vi "Savecalil_data.vi"(8 "错误输入（无错误）":errorcluster, 11 "PDLSTS":refnum<k24>) -> (0 "错误输出":errorcluster)   [LabVIEW 2017]
doc: "// Save Calculated IL (Cancel for SOP wavelength dependence)\n // This method must be run after the PDL Calculation"
uses:
  D:/test/PDLSTS/LV_PDL_Sample/DLL/STSProcess.dll
  DLL/STSProcess.dll
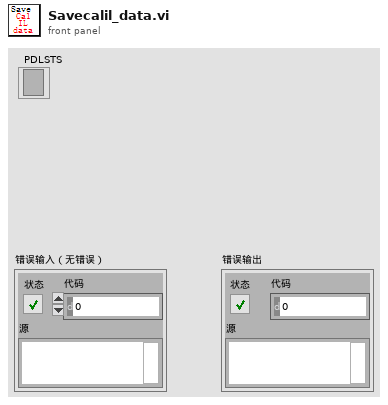
[diagram p1: front panel]
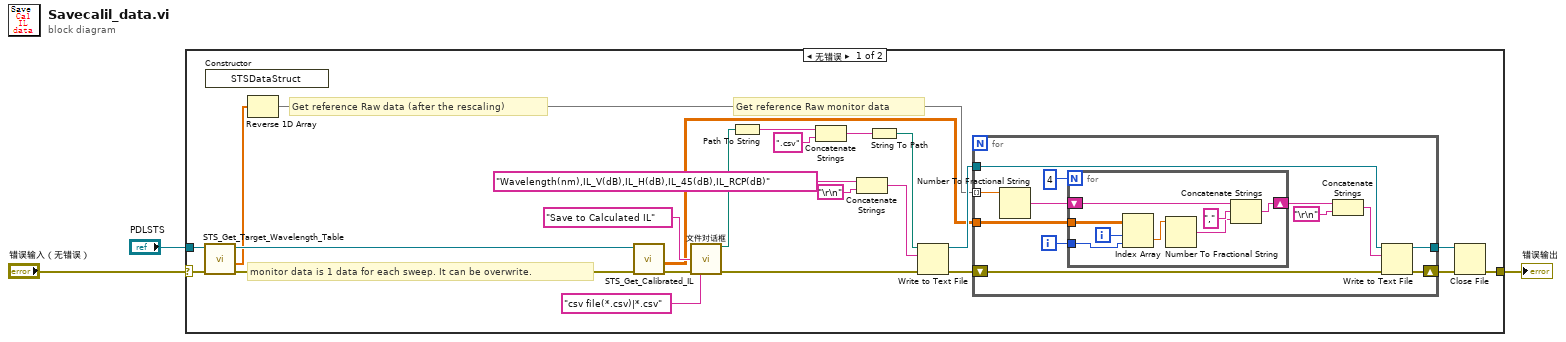
[diagram p0: block diagram]
diagram:
  n1 = case shown="无错误" "错误输入（无错误）" {
    selector: "错误输入（无错误）" -> [w26 w48]
    tunnel: [w27 w48] -> w3
    tunnel: "PDLSTS" -> [w25 _]
    frame No Error {
      # "Get reference Raw monitor data"
      # "monitor data is 1 data for each sweep. It can be overwrite."
      # "Get reference Raw data (after the rescaling)"
      n2 = call "STS_Get_Target_Wavelength_Table.vi"("错误输入（无错误）"=w26, ".NET引用句柄输入"=w25) -> ("error out"=w10:errorcluster, "wavelengths"=w5:dbl[], "引用输出"=w11:refnum<k24>)  [unwired: 7 in]
      n3 = constructor class="STSDataStruct"() -> ()  [unwired: 3 in, 3 out]
      n4 = Reverse 1D Array(array=w5) -> (reversed array=w4:dbl[])
      n5 = call "STS_Get_Calibrated_IL.vi"("错误输入（无错误）"=w10, ".NET引用句柄输入"=w11) -> ("error out"=w8:errorcluster, "calibratedIL"=w6:sgl[][])  [unwired: 7 in, 1 out]
      n6 = call "文件对话框"("default name"="Save to Calculated IL" ("字符串"), "error in"=w8, "pattern (all files)"="csv file(*.csv)|*.csv") -> ("selected path"=w13:path, "error out"=w21:errorcluster)  [unwired: 9 in, 2 out]
      n7 = Path To String(path=w13) -> (string=w12:string)
      n8 = Concatenate Strings(w12, ".csv" ("名称或相对路径")) -> (w19:string)
      n9 = Concatenate Strings("Wavelength(nm),IL_V(dB),IL_H(dB),IL_45(dB),IL_RCP(dB)", "\r\n") -> (w23:string)
      n10 = String To Path(string=w19) -> (path=w18:path)
      n11 = Write to Text File(file (use dialog)=w18, text=w23, error in=w21) -> (refnum out=w16:refnum<file>, error out=w7:errorcluster)  [unwired: 1 in, 1 out]
      n12 = for {
        tunnel: w4 -> [w39] mode=indexing
        tunnel: w16 -> [w34]
        tunnel: [w33] -> w15
        shift-right: [w36] -> w14
        shift-left: w7 -> [w37]
        tunnel: w6 -> [w28]
        i -> [w30]
        n13 = Number To Fractional String(number=w39) -> (F-format string=w38:string)  [unwired: 3 in]
        n14 = for {
          N: 4 -> [_]
          tunnel: w28 -> [w47]
          tunnel: w30 -> [w46]
          shift-right: [w42] -> w31
          shift-left: w38 -> [w43]
          i -> [w45]
          n15 = Index Array(array=w47, index (row)=w45, index (col)=w46) -> (element=w44:sgl)
          n16 = Number To Fractional String(number=w44) -> (F-format string=w40:string)  [unwired: 3 in]
          n17 = Concatenate Strings(w43, "," ("字符串"), w40) -> (w42:string)
        }
        n18 = Concatenate Strings(w31, "\r\n") -> (w35:string)
        n19 = Write to Text File(file (use dialog)=w34, text=w35, error in=w37) -> (refnum out=w33:refnum<file>, error out=w36:errorcluster)  [unwired: 1 in, 1 out]
      }
      n20 = Close File(refnum=w15, error in=w14) -> (error out=w27:errorcluster)  [unwired: 1 out]
    }
    frame Error {
    }
  }
  "错误输出" <- w3
